vi "setT.vi"(0 "ITCSignal":T1={"ITC"=0, "Signal"=enum."Sensor 3"}, 1 "T target [K]":dbl=1.8, 2 "upper limit":dbl=310.0, 3 "lower limit":dbl=0.25, 4 "Switch off?":bool) -> (5 "ITCSignal 2":T1={"ITC"=0, "Signal"=enum."Sensor 3"}, 6 "coerced(x)":dbl)   [LabVIEW 2011]
uses:
  Kelvinox drivers/ITCAPPS - Copie.LLB/ITCSignal.ctl
  Kelvinox drivers/ITCAPPS.LLB/ITCSignals.ctl
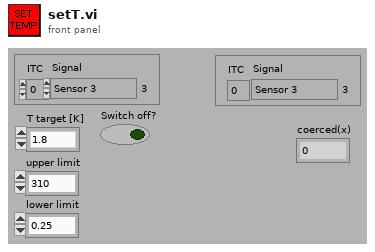
[diagram p1: front panel]
types:
  T1 = typedef "ITCSignal.ctl" = cluster{"ITC":u16, "Signal":T2}
  T2 = typedef "ITCSignals.ctl" = enum16{"Setpoint", "Sensor 1", "Sensor 2", "Sensor 3", "Needle Valve %", "Heater %"}
  T3 = typedef "ITCSetup.ctl" = cluster{"Description":string, "IO Info":T4}
  T4 = typedef "ITCIO.ctl" = cluster{"Address":T5, "Version":T6, "Ch 1 dec places":i16, "Ch 2 dec places":i16, "Ch 3 dec places":i16, "Ch1 Name":string, "Ch2 Name":string, "Ch3 Name":string}
  T5 = typedef "OxfordAddress.ctl" = cluster{"Com Port":i32, "ISOBUS Address":i32, "GPIB Address":i16, "Communication":enum16{"RS232", "ISOBUS", "GPIB", "Gateway"}}
  T6 = typedef "ITCVersion.ctl" = enum16{"ITC502", "ITC503", "ITC601"}
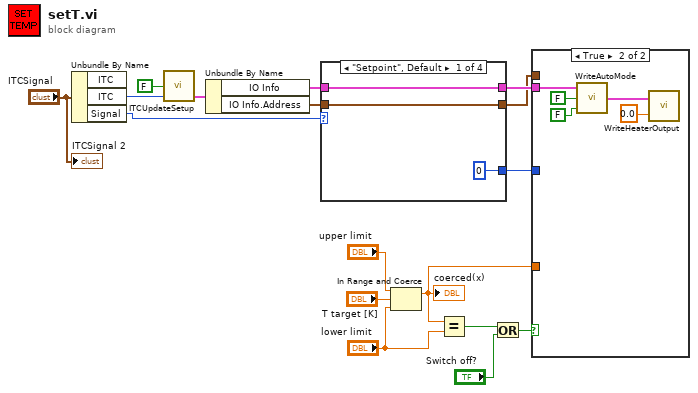
[diagram p0: block diagram]
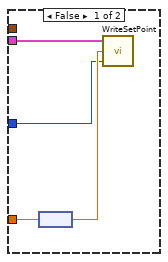
[diagram p2: hidden frame]
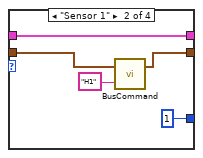
[diagram p3: hidden frame]
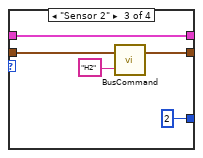
[diagram p4: hidden frame]
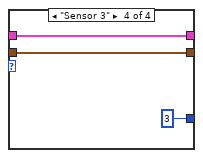
[diagram p5: hidden frame]
diagram:
  n1 = Unbundle By Name("ITCSignal") -> ("ITC"=w15:u16, "Signal"=w12:T2)  [unwired: 1 out]
  n2 = call "ITCUpdateSetup.vi"("Index"=w15, "Write to disk?"=FALSE) -> ("ITC Setup"=w14:T3)  [unwired: 2 in, 1 out]
  n3 = Unbundle By Name(w14) -> ("IO Info"=w13:T4, "IO Info.Address"=w2:T5)
  n4 = case shown="\"Setpoint\", Default" w12 {
    tunnel: w13 -> [w20 w24 w29 w32]
    tunnel: [w20 w24 w29 w32] -> w17
    tunnel: [i16 0 ("Control Channel") i16 1 ("Control Channel") i16 2 ("Control Channel") i16 3 ("Control Channel")] -> w3
    tunnel: w2 -> [w18 w22 w28 w31]
    tunnel: [w18 w21 w26 w31] -> w1
    frame "Setpoint", Default {
    }
    frame "Sensor 1" {
      n5 = call "BusCommand.vi"("Command"="H1", "Instrument address (in)"=w22) -> ("Instrument address (out)"=w21:T5)  [unwired: 1 out]
    }
    frame "Sensor 2" {
      n6 = call "BusCommand.vi"("Command"="H2", "Instrument address (in)"=w28) -> ("Instrument address (out)"=w26:T5)  [unwired: 1 out]
    }
    frame "Sensor 3" {
    }
  }
  n7 = In Range and Coerce(upper limit="upper limit", x="T target [K]", lower limit="lower limit") -> (coerced(x)=w4:dbl)  [unwired: 1 out]
  "coerced(x)" <- w4
  n8 = Equal?(x=w4, y="lower limit") -> (x = y?=w6:bool)
  n9 = Or(x=w6, y="Switch off?") -> (x .or. y?=w5:bool)
  n10 = case shown="True" w5 {
    tunnel: w17 -> [w36 w38]
    tunnel: w4 -> [w35 _]
    tunnel: w3 -> [w34 _]
    tunnel: w1 -> [_ _]
    frame False {
      n11 = node(w35) -> (w37:dbl[unit])
      n12 = call "WriteSetPoint.vi"("Control Ch"=w34, "Set point"=w37, "IO Info"=w36) -> ()  [unwired: 1 out]
    }
    frame True {
      n13 = call "WriteAutoMode.vi"("Auto Needle Valve"=FALSE, "Auto Heat"=FALSE, "ITC IO Info"=w38) -> ("ITC IO Info"=w40:T4)
      n14 = call "WriteHeaterOutput.vi"("Heater Output (%)"=0.0, "ITC IO Info"=w40) -> ()  [unwired: 1 in, 1 out]
    }
  }
  "ITCSignal 2" <- "ITCSignal"
